vi "Get Colleague Name.vi"(8 "error in (no error)":errorcluster caption="错误输入（无错误）", 11 "同事（抽象）输入":refnum<class "Colleague.lvclass">) -> (0 "error out":errorcluster caption="错误输出", 2 "同事名称":string, 3 "同事（抽象）输出":refnum<class "Colleague.lvclass">)   [LabVIEW 2011, in "Colleague.lvclass"]
uses:
  Colleague.lvclass
  Colleague.lvclass/Colleague.ctl
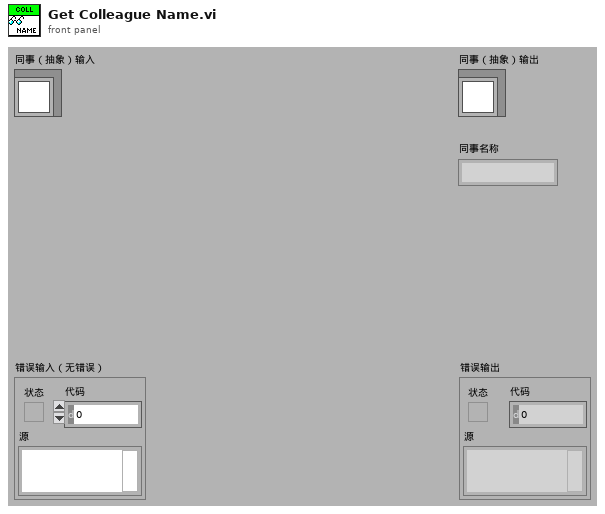
[diagram p1: front panel]
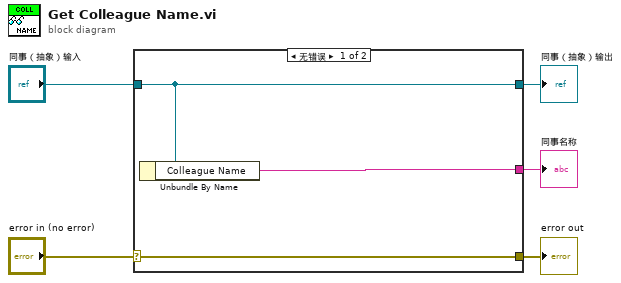
[diagram p0: block diagram]
diagram:
  n1 = case shown="无错误" "error in (no error)" {
    selector: "error in (no error)" -> [w8 w9]
    tunnel: [w8 w9] -> w4
    tunnel: [w7 w10] -> w2
    tunnel: "同事（抽象）输入" -> [w7 w10]
    tunnel: [w6 _] -> w1
    frame No Error {
      n2 = Unbundle By Name(w7) -> ("Colleague Name"=w6:string)
    }
    frame Error {
    }
  }
  "error out" <- w4
  "同事（抽象）输出" <- w2
  "同事名称" <- w1
